vi "ConvertXScaleTimes.vi"(3 "InputKnob":u16, 4 "Time2Knob?":bool=TRUE, 5 "InputTime":dbl format="%#_13g") -> (0 "OutputTime":dbl format="%#_13g", 1 "OutputKnob":u16)   [LabVIEW 2014, in "CS++ScopeGui.lvlib" / "CS++ScopeGui.lvclass"]
doc: "Small conversion needed inside the ActorCore"
uses:
  CS++ScopeGui.lvclass
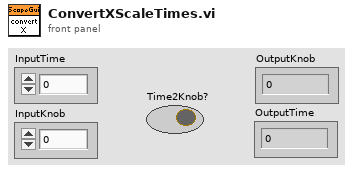
[diagram p1: front panel]
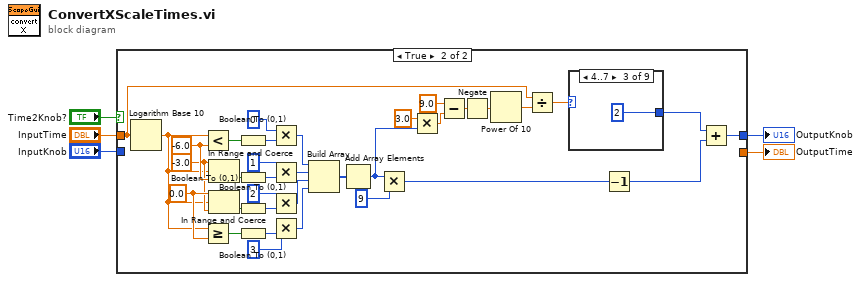
[diagram p0: block diagram]
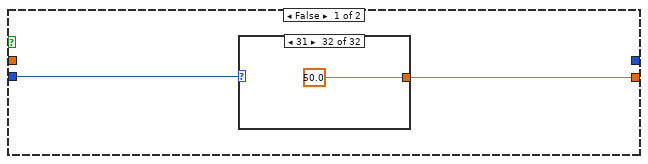
[diagram p2: hidden frame]
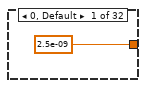
[diagram p3: hidden frame]
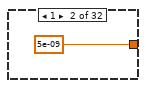
[diagram p4: hidden frame]
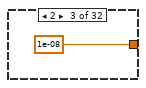
[diagram p5: hidden frame]
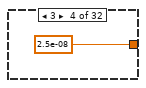
[diagram p6: hidden frame]
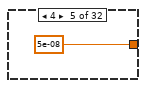
[diagram p7: hidden frame]
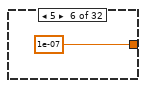
[diagram p8: hidden frame]
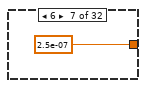
[diagram p9: hidden frame]
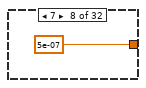
[diagram p10: hidden frame]
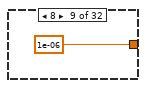
[diagram p11: hidden frame]
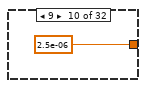
[diagram p12: hidden frame]
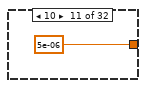
[diagram p13: hidden frame]
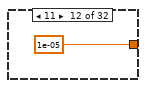
[diagram p14: hidden frame]
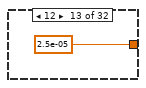
[diagram p15: hidden frame]
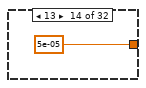
[diagram p16: hidden frame]
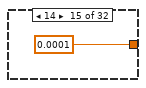
[diagram p17: hidden frame]
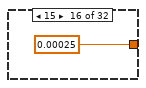
[diagram p18: hidden frame]
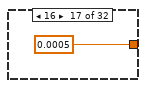
[diagram p19: hidden frame]
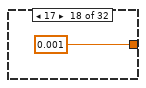
[diagram p20: hidden frame]
diagram:
  n1 = case shown="True" "Time2Knob?" {
    tunnel: "InputTime" -> [_ w43]
    tunnel: [_ w53] -> w3
    tunnel: "InputKnob" -> [w7 _]
    tunnel: [w6 _] -> w1
    frame False {
      n2 = case shown="31" w7 {
        tunnel: [2.5e-09 5e-09 1e-08 2.5e-08 5e-08 1e-07 2.5e-07 5e-07 1e-06 2.5e-06 5e-06 1e-05 2.5e-05 5e-05 0.0001 0.00025 0.0005 0.001 0.0025 0.005 0.01 0.025 0.05 0.1 0.25 0.5 1.0 2.5 5.0 10.0 25.0 50.0] -> w6
        frame 0, Default {
        }
        frame 1 {
        }
        frame 2 {
        }
        frame 3 {
        }
        frame 4 {
        }
        frame 5 {
        }
        frame 6 {
        }
        frame 7 {
        }
        frame 8 {
        }
        frame 9 {
        }
        frame 10 {
        }
        frame 11 {
        }
        frame 12 {
        }
        frame 13 {
        }
        frame 14 {
        }
        frame 15 {
        }
        frame 16 {
        }
        frame 17 {
        }
        frame 18 {
        }
        frame 19 {
        }
        frame 20 {
        }
        frame 21 {
        }
        frame 22 {
        }
        frame 23 {
        }
        frame 24 {
        }
        frame 25 {
        }
        frame 26 {
        }
        frame 27 {
        }
        frame 28 {
        }
        frame 29 {
        }
        frame 30 {
        }
        frame 31 {
        }
      }
    }
    frame True {
      w73 = 0.0 ("upper limit")
      w57 = -3.0 ("y")
      w74 = -6.0 ("y")
      n3 = Logarithm Base 10(1:w43) -> (0:w46:dbl)
      n4 = Less?(x=w46, y=w74) -> (x < y?=w72:bool)
      n5 = Greater Or Equal?(x=w46, y=w73) -> (x >= y?=w69:bool)
      n6 = In Range and Coerce(upper limit=w57, x=w46, lower limit=w74) -> (In Range?=w71:bool)  [unwired: 1 out]
      n7 = In Range and Coerce(upper limit=w73, x=w46, lower limit=w57) -> (In Range?=w70:bool)  [unwired: 1 out]
      n8 = Boolean To (0,1)(Boolean=w72) -> (0, 1=w65:i16)
      n9 = Boolean To (0,1)(Boolean=w71) -> (0, 1=w66:i16)
      n10 = Boolean To (0,1)(Boolean=w70) -> (0, 1=w67:i16)
      n11 = Boolean To (0,1)(Boolean=w69) -> (0, 1=w68:i16)
      n12 = Multiply(x=i16 0, y=w65) -> (x*y=w61:i16)
      n13 = Multiply(x=i16 1, y=w66) -> (x*y=w60:i16)
      n14 = Multiply(x=i16 2, y=w67) -> (x*y=w59:i16)
      n15 = Multiply(x=i16 3, y=w68) -> (x*y=w58:i16)
      n16 = Build Array(w61, w60, w59, w58) -> (w55:i16[])
      n17 = Add Array Elements(numeric array=w55) -> (sum=w42:i16)
      n18 = Multiply(x=w42, y=i16 9) -> (x*y=w41:i16)
      n19 = Multiply(x=3.0, y=w42) -> (x*y=w50:dbl)
      n20 = Subtract(x=9.0, y=w50) -> (x-y=w49:dbl)
      n21 = Negate(x=w49) -> (-x=w48:dbl)
      n22 = Power Of 10(x=w48) -> (10^x=w47:dbl)
      n23 = Divide(x=w43, y=w47) -> (x/y=w45:dbl)
      n24 = case shown="4..7" w45 {
        tunnel: [0 1 2 3 4 5 6 7 8] -> w44
        frame ..1 {
        }
        frame 2, 3 {
        }
        frame 4..7 {
        }
        frame 8..15 {
        }
        frame 16..30 {
        }
        frame 31..70 {
        }
        frame 71..150 {
        }
        frame 151..300 {
        }
        frame 301.. {
        }
      }
      n25 = Decrement(x=w41) -> (x-1=w40:i16)
      n26 = Add(x=w44, y=w40) -> (x+y=w53:i32)
    }
  }
  "OutputKnob" <- w3
  "OutputTime" <- w1
